vi "Toma_A.vi"() -> ()   [LabVIEW 2017]
uses:
  Maquina_de_Estados_Type_Def.ctl
  Cluster_de_Datos.ctl
  <vilib>/DAQmx/read.llb/DAQmx Read (Analog 1D DBL 1Chan NSamp).vi
  <vilib>/DAQmx/create/channels.llb/DAQmx Create Channel (AI-Voltage-Basic).vi
  <vilib>/DAQmx/configure/timing.llb/DAQmx Timing (Sample Clock).vi
  <vilib>/DAQmx/miscellaneous.llb/DAQmx Fill In Error Info.vi
  <vilib>/imath/engines/lvmath2/RunTimeEngine/BuiltInFunctions/length/NIMS_length(GV).vi
  <instcachedir>/0/NIMS_length(GV)_08A3D13377FD4E4B96F5795FBF3698FA.lvgen/NIMS_length(GV)_08A3D13377FD4E4B96F5795FBF3698FA_000.vi
  <vilib>/imath/engines/lvmath2/RunTimeEngine/IndexReplace/NIMS V(S)=S.vi
  <instcachedir>/0/NIMS V(S)=S_3F4D177D41884A9C969E5FA0B22E4B28.lvgen/NIMS V(S)=S_3F4D177D41884A9C969E5FA0B22E4B28_003.vi
  <vilib>/imathl/engines/lvmath/Functions/Error Handling/Create Error.vi
  <vilib>/imath/engines/lvmath2/RunTimeEngine/RangeToken/NIMS_Range_R2 - Integer.vi
  <instcachedir>/0/NIMS_Range_R2 - Integer_B2C3C6B11D0E4F789E1772ACB483EB02.lvgen/NIMS_Range_R2 - Integer_B2C3C6B11D0E4F789E1772ACB483EB02_000.vi
  <vilib>/imath/engines/lvmath2/RunTimeEngine/CommandStatement/MC_CommandStatement_break.vi
  <vilib>/imath/engines/lvmath2/RunTimeEngine/IndexRead/NIMS V(S).vi
  <instcachedir>/0/NIMS V(S)_0488751826AF41519A22953C041130DC.lvgen/NIMS V(S)_0488751826AF41519A22953C041130DC_000.vi
  <instcachedir>/0/NIMS V(S)=S_3F4D177D41884A9C969E5FA0B22E4B28.lvgen/NIMS V(S)=S_3F4D177D41884A9C969E5FA0B22E4B28_000.vi
  <vilib>/imath/engines/lvmath2/RunTimeEngine/ErrorHandling/NIMS_Create Error From Enums.vi
  <vilib>/imath/engines/lvmath2/RunTimeEngine/NodeEndStatement/NIMS_NodeEndStatement_Output.vi
  <instcachedir>/0/NIMS_NodeEndStatement_Output_53EC0D466D134D7ABD903AC30B43404B.lvgen/NIMS_NodeEndStatement_Output_53EC0D466D134D7ABD903AC30B43404B_005.vi
  <vilib>/imath/engines/lvmath2/RunTimeEngine/ErrorHandling/NIMS_Finalize Error.vi
  <vilib>/addons/_office/excel.llb/Excel Get Data (i32).vi
  <vilib>/addons/_office/excel.llb/Excel Easy Table (num).vi
  <vilib>/Utility/NIReport.llb/NI_report.lvclass
  <vilib>/Utility/NIReport.llb/Excel/NI_Excel.lvclass
  <vilib>/addons/_office/NI_ReportGenerationToolkit.lvlib
panel:
  in  "Ruta del Reporte":path
  in  "Ruta_Logo_IPN":path
  in  "Ruta_Logo_Upiita":path=path "C:/Users/LuisFernando/Documents/UPIITA/8vo semestre/Instrumentacion Virtual Aplicada/DAQ/Logo_Upiita.bmp"
  in  "Actualizar Rutas":bool
  in  "Calificacion":dbl
  in  "Grupo":string
  in  "Unidad de Aprendizaje":string
  in  "Leer Senal":bool
  in  "stop":bool
  in  "Comentarios":string
  out "Hora":string
  out "Fecha":string
  in  "Nombre (s):":string(combo)
  in  "Tab Control":enum32{"Función", "Derivada", "Integral"}(tab)
  out "Señal de Entrada M":dbl[](graph)
  out "Señal de Entrada":cluster{dbl[], "data":dbl[]}(graph)
  out "Derivada M":dbl[](graph)
  out "Derivada":cluster{"Tiempo":dbl[], "Diff":dbl[]}(graph)
  out "Integral M":dbl[](graph)
  out "Integral":cluster{"Tiempo":dbl[], "Integral":dbl[]}(graph)
  out "Escudo 2":picture
  out "Escudo_1":picture
  # "INSTITUTO POLITECNICO NACIONAL"
  # "Unidad Profesional Interdisciplinaria en\nIngenieria y Tecnologias Avanzadas"
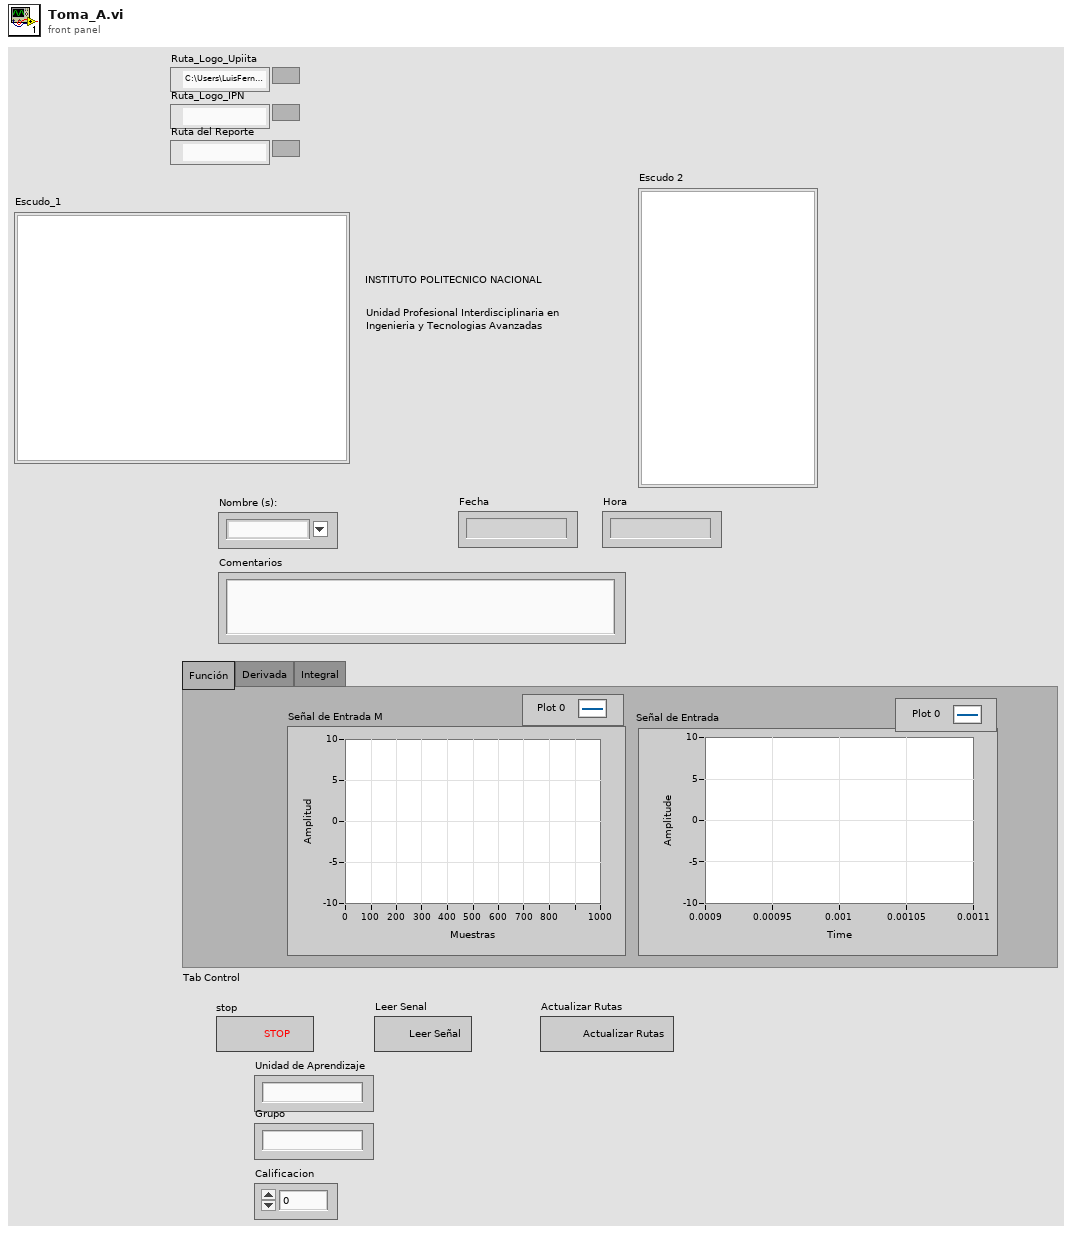
[diagram p1: front panel]
types:
  T1 = typedef "Cluster_de_Datos.ctl" = cluster{"Error":errorcluster, "Ruta_Logo_Upiita":path, "Ruta_Logo_IPN":path, "Señal de Entrada":dbl[], "Derivada":dbl[], "Integral":dbl[], "Muestras":i32, "Frecuencia de Muestreo":dbl, "Tiempo":dbl[], "dt":dbl, "Ruta del Reporte":path, "Numero de Hoja":u32}
  T2 = typedef "Maquina_de_Estados_Type_Def.ctl" = enum16{"Configuracion Inicial", "Espera", "Leer Senal", "Derivar", "Integrar", "Leer Datos de Usuario", "Salir"}
  T3 = enum16{"maximized", "minimized", "normal", "no change"}
  T4 = enum16{"Standard Report", "HTML", "Word", "Excel"}
  T5 = typedef "imagedata.ctl" = cluster{"image type":i32, "image depth":i32, "image":u8[], "mask":u8[], "colors":u32[], "Rectangle":cluster{"left":i16, "top":i16, "right":i16, "bottom":i16}}
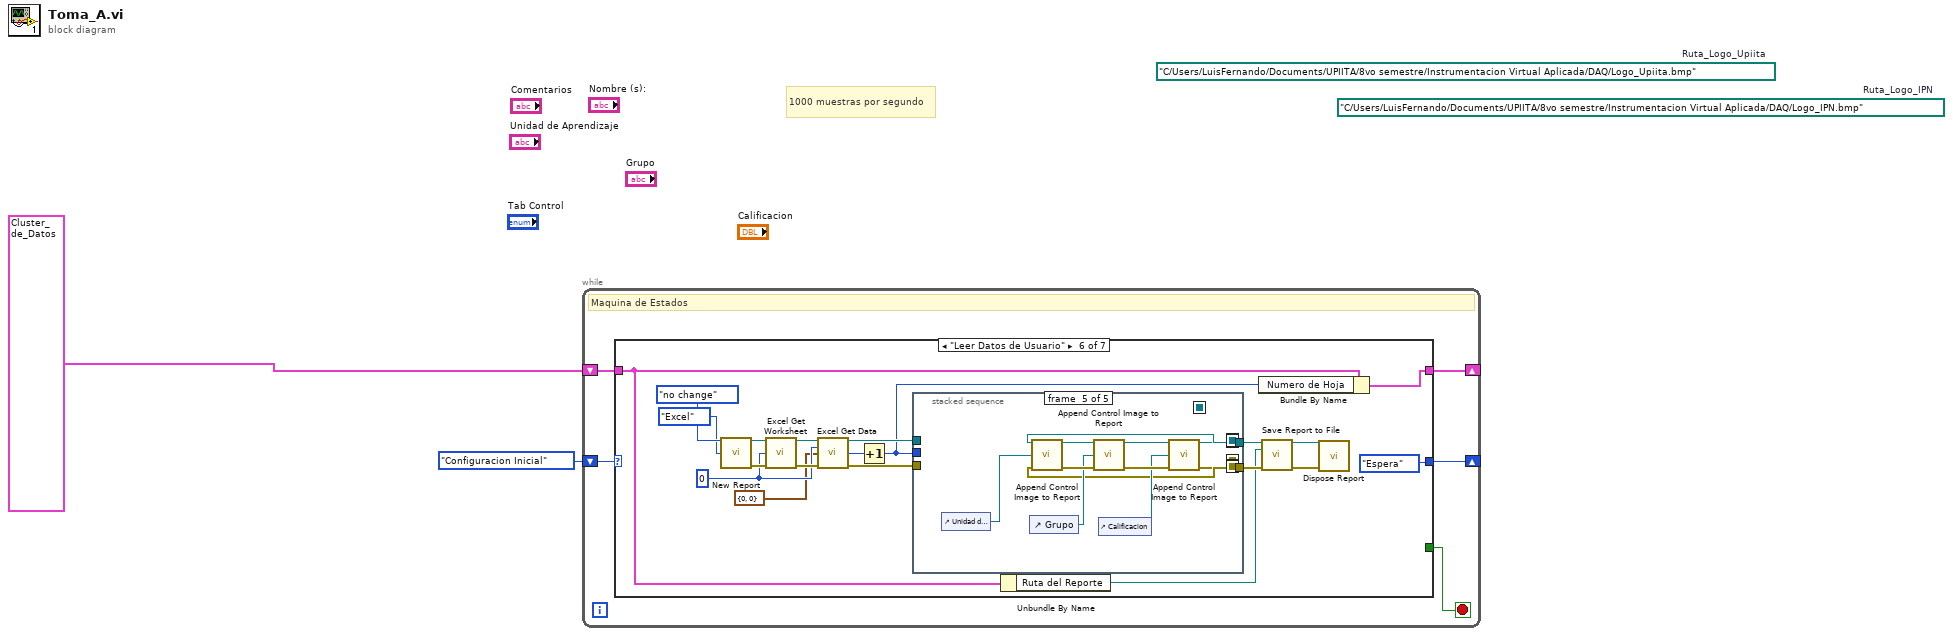
[diagram p0: block diagram]
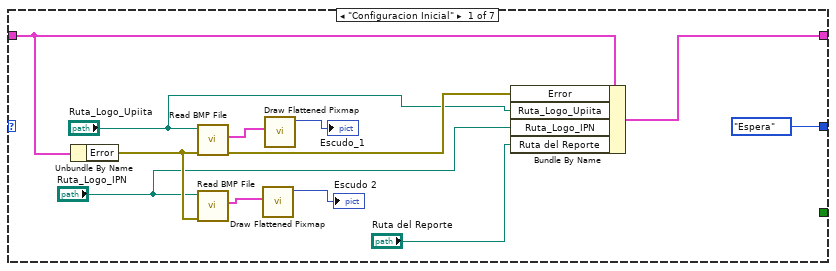
[diagram p2: hidden frame]
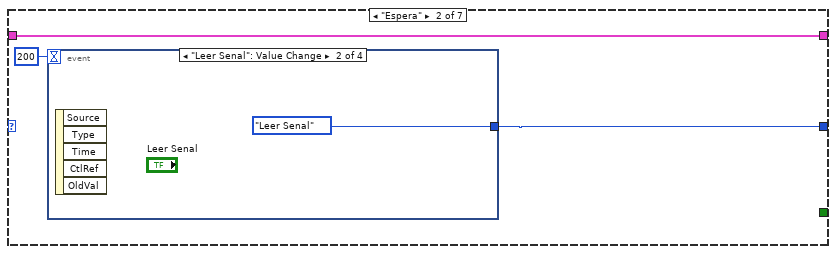
[diagram p3: hidden frame]
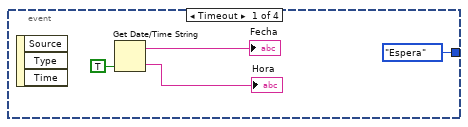
[diagram p4: hidden frame]
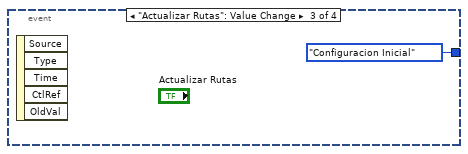
[diagram p5: hidden frame]
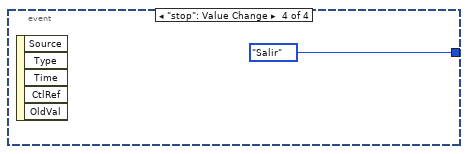
[diagram p6: hidden frame]
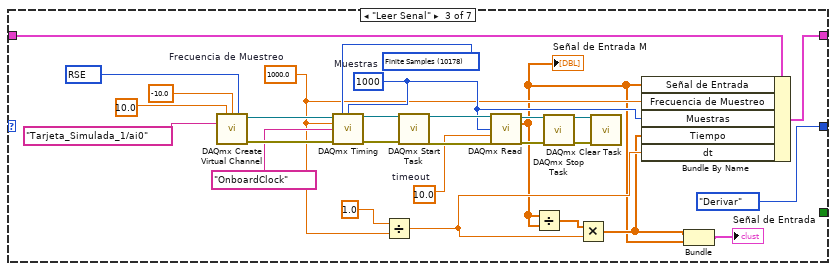
[diagram p7: hidden frame]
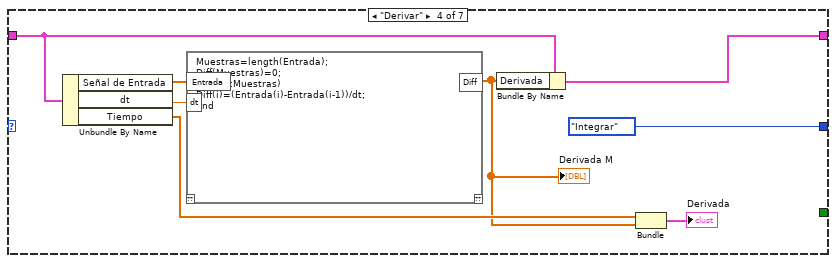
[diagram p8: hidden frame]
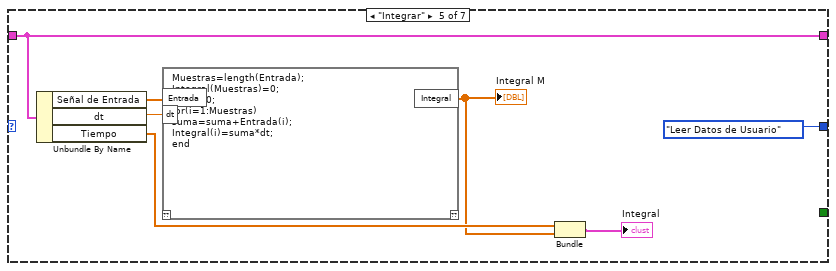
[diagram p9: hidden frame]
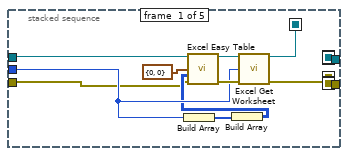
[diagram p10: hidden frame]
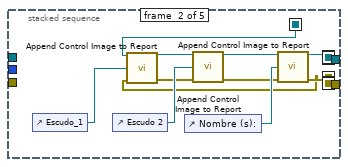
[diagram p11: hidden frame]
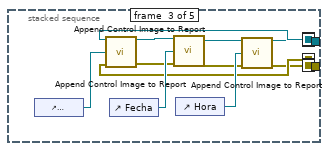
[diagram p12: hidden frame]
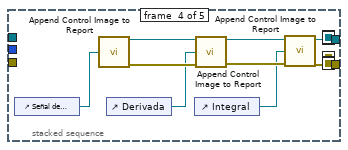
[diagram p13: hidden frame]
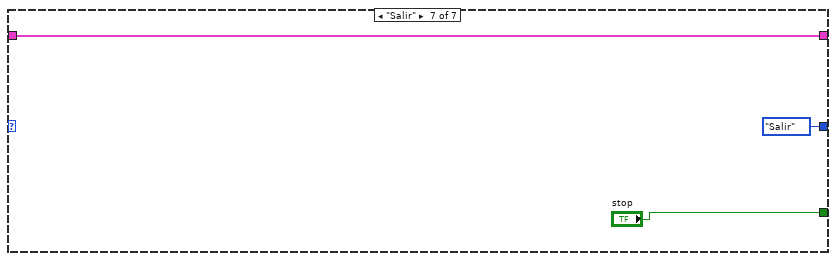
[diagram p14: hidden frame]
diagram:
  (unwired) path "C:/Users/LuisFernando/Documents/UPIITA/8vo semestre/Instrumentacion Virtual Aplicada/DAQ/Logo_IPN.bmp"  # Ruta_Logo_IPN
  (unwired) path "C:/Users/LuisFernando/Documents/UPIITA/8vo semestre/Instrumentacion Virtual Aplicada/DAQ/Logo_Upiita.bmp"  # Ruta_Logo_Upiita
  # "1000 muestras por segundo"
  n1 = while {
    shift-right: [w6] -> _
    shift-left: Maquina_de_Estados_Type_Def."Configuracion Inicial" -> [w7]
    shift-right: [w4] -> _
    shift-left: T1 {"Error"={"status"=FALSE, "code"=0, "source"=""}, "Ruta_Logo_Upiita"=path "C:/Users/LuisFernando/Documents/UPIITA/8vo semestre/Instrumentacion Virtual Aplicada/DAQ/Logo_Upiita.bmp", "Ruta_Logo_IPN"=path "C:/Users/LuisFernando/Documents/UPIITA/8vo semestre/Instrumentacion Virtual Aplicada/DAQ/Logo_IPN.bmp", "Señal de Entrada"=[], "Derivada"=[], "Integral"=[], "Muestras"=1000, "Frecuencia de Muestreo"=10.0, "Tiempo"=[], "dt"=1000.0, "Ruta del Reporte"=path "C:/Users/LuisFernando/Documents/UPIITA/8vo semestre/Instrumentacion Virtual Aplicada/DAQ/Logo_IPN.bmp", "Numero de Hoja"=0} -> [w5]
    stop <- w3 stop-if-true
    # "Maquina de Estados"
    n2 = case shown="\"Leer Datos de Usuario\"" w7 {
      tunnel: [Maquina_de_Estados_Type_Def."Espera" w21 Maquina_de_Estados_Type_Def."Derivar" Maquina_de_Estados_Type_Def."Integrar" Maquina_de_Estados_Type_Def."Leer Datos de Usuario" Maquina_de_Estados_Type_Def."Espera" Maquina_de_Estados_Type_Def."Salir"] -> w6
      tunnel: w5 -> [w15 w22 w39 w63 w182 w318 w393]
      tunnel: [w17 w22 w38 w62 w182 w335 w393] -> w4
      tunnel: [_ _ _ _ _ _ "stop"] -> w3
      frame "Configuracion Inicial" {
        n3 = Unbundle By Name(w15) -> ("Error"=w13:errorcluster)
        n4 = call <vilib>:"Read BMP File.vi"("error in (no error)"=w13, "path to BMP file"="Ruta_Logo_Upiita") -> ("error out"=w16:errorcluster, "image data"=w18:T5)  [unwired: 7 in, 1 out]
        n5 = call <vilib>:"Read BMP File.vi"("error in (no error)"=w13, "path to BMP file"="Ruta_Logo_IPN") -> ("image data"=w14:T5)  [unwired: 7 in, 2 out]
        n6 = call <vilib>:"Draw Flattened Pixmap.vi"("image data"=w14) -> ("new picture"=→"Escudo 2":picture)  [unwired: 8 in]
        n7 = call <vilib>:"Draw Flattened Pixmap.vi"("image data"=w18) -> ("new picture"=→"Escudo_1":picture)  [unwired: 8 in]
        n8 = Bundle By Name(cluster=w15, "Error"=w16, "Ruta_Logo_Upiita"="Ruta_Logo_Upiita", "Ruta_Logo_IPN"="Ruta_Logo_IPN", "Ruta del Reporte"="Ruta del Reporte") -> (w17:T1)
      }
      frame "Espera" {
        n9 = event shown="[1] \"Leer Senal\": Value Change" {
          selector: _ -> [_ _ _ _]
          dyn-events: _ -> [_ _ _ _]
          timeout: 200 -> [_ _ _ _]
          tunnel: [Maquina_de_Estados_Type_Def."Espera" Maquina_de_Estados_Type_Def."Leer Senal" Maquina_de_Estados_Type_Def."Configuracion Inicial" Maquina_de_Estados_Type_Def."Salir"] -> w21
          event Timeout {
            n10 = event-data() -> ()  [unwired: 1 in, 3 out]
            n11 = Get Date/Time String(want seconds? (F)=TRUE) -> (date string=→"Fecha":string, time string=→"Hora":string)  [unwired: 2 in]
          }
          event "Leer Senal": Value Change {
            n12 = event-data() -> ()  [unwired: 1 in, 5 out]
          }
          event "Actualizar Rutas": Value Change {
            n13 = event-data() -> ()  [unwired: 1 in, 5 out]
          }
          event "stop": Value Change {
            n14 = event-data() -> ()  [unwired: 1 in, 5 out]
          }
        }
      }
      frame "Leer Senal" {
        w46 = 10.0  # timeout
        w41 = 10083 items=["Default"=-1, "RSE"=10083, "NRSE"=10078, "Differential"=10106, "Pseudodifferential"=12529] ("input terminal configuration")
        w35 = 1000.0  # Frecuencia de Muestreo
        w37 = 1000  # Muestras
        w45 = 10178 items=["Finite Samples"=10178, "Continuous Samples"=10123, "Hardware Timed Single Point"=12522] ("sample mode")
        n15 = call-poly <vilib>:"DAQmx Create Virtual Channel.vi"("maximum value"=10.0, "minimum value"=-10.0, "input terminal configuration"=w41, "physical channels"=tag "Tarjeta_Simulada_1/ai0") -> ("task out"=w48:refnum<k21>, "error out"=w47:errorcluster)  [unwired: 10 in]
        n16 = call-poly <vilib>:"DAQmx Timing.vi"("task/channels in"=w48, "sample mode"=w45, "samples per channel"=w37, "rate"=w35, "source"=tag "OnboardClock", "error in"=w47) -> ("task out"=w49:refnum<k21>, "error out"=w50:errorcluster)  [unwired: 8 in]
        n17 = Divide(x=1.0, y=w35) -> (x/y=w33:dbl)
        n18 = call <vilib>:"DAQmx Start Task.vi"("task/channels in"=w49, "error in"=w50) -> ("task out"=w51:refnum<k21>, "error out"=w52:errorcluster)  [unwired: 12 in]
        n19 = call-poly <vilib>:"DAQmx Read.vi"("task/channels in"=w51, "number of samples per channel"=w37, "timeout"=w46, "error in"=w52) -> ("task out"=w53:refnum<k21>, "data"=w31:dbl[], "error out"=w54:errorcluster)  [unwired: 9 in]
        "Señal de Entrada M" <- w31
        n20 = Divide(x=w31, y=w31) -> (x/y=w34:dbl[])
        n21 = call <vilib>:"DAQmx Stop Task.vi"("task/channels in"=w53, "error in"=w54) -> ("task out"=w55:refnum<k21>, "error out"=w56:errorcluster)  [unwired: 12 in]
        n22 = Multiply(x=w34, y=w33) -> (x*y=w32:dbl[])
        n23 = call <vilib>:"DAQmx Clear Task.vi"("task in"=w55, "error in"=w56) -> ()  [unwired: 13 in, 1 out]
        n24 = Bundle By Name(cluster=w39, "Señal de Entrada"=w31, "Frecuencia de Muestreo"=w35, "Muestras"=w37, "Tiempo"=w32, "dt"=w33) -> (w38:T1)
        n25 = Bundle(w32, "data"=w31) -> (→"Señal de Entrada":cluster{dbl[], "data":dbl[]})  [unwired: 1 in]
      }
      frame "Derivar" {
        n26 = Unbundle By Name(w63) -> ("Señal de Entrada"=w64:dbl[], "dt"=w61:dbl, "Tiempo"=w59:dbl[])
        n27 = mathscript code="Muestras=length(Entrada);\nDiff(Muestras)=0;\nfor(i=2:Muestras)\nDiff(i)=(Entrada(i)-Entrada(i-1))/dt;\nend"("Entrada"=w64, "dt"=w61) -> ("Diff"=w58:dbl[])  [unwired: 1 in, 1 out]
        "Derivada M" <- w58
        n28 = Bundle By Name(cluster=w63, "Derivada"=w58) -> (w62:T1)
        n29 = Bundle("Tiempo"=w59, "Diff"=w58) -> (→"Derivada":cluster{"Tiempo":dbl[], "Diff":dbl[]})  [unwired: 1 in]
      }
      frame "Integrar" {
        n30 = Unbundle By Name(w182) -> ("Señal de Entrada"=w181:dbl[], "dt"=w180:dbl, "Tiempo"=w179:dbl[])
        n31 = mathscript code="Muestras=length(Entrada);\nIntegral(Muestras)=0;\nsuma=0;\nfor(i=1:Muestras)\nsuma=suma+Entrada(i);\nIntegral(i)=suma*dt;\nend"("Entrada"=w181, "dt"=w180) -> ("Integral"=w177:dbl[])  [unwired: 1 in, 1 out]
        "Integral M" <- w177
        n32 = Bundle("Tiempo"=w179, "Integral"=w177) -> (→"Integral":cluster{"Tiempo":dbl[], "Integral":dbl[]})  [unwired: 1 in]
      }
      frame "Leer Datos de Usuario" {
        w323 = 0 ("worksheet index (0)")
        n33 = call <vilib>:"New Report.vi"("window state (normal)"=T3."no change", "report type"=T4."Excel") -> ("report out"=w332:refnum<class "NI_report.lvclass">, "error out"=w331:errorcluster)  [unwired: 12 in]
        n34 = call <vilib>:"Excel Get Worksheet.vi"("report in"=w332, "worksheet index (0)"=w323, "error in (no error)"=w331) -> ("report out"=w330:refnum<class "NI_report.lvclass">, "error out"=w329:errorcluster)  [unwired: 11 in]
        n35 = call-poly <vilib>:"Excel Get Data.vi"("report in"=w330, "data type"=w323, "start (0, 0)"=cluster{"start row":i32, "start column":i32} {"start row"=0, "start column"=0}, "error in (no error)"=w329) -> ("report out"=w333:refnum<class "NI_report.lvclass">, "data"=w328:i32, "error out"=w334:errorcluster)  [unwired: 9 in]
        n36 = Increment(x=w328) -> (x+1=w319:i32)
        n37 = stacked-sequence {
          seq-local: [w344 _ _ _ _] -> [_ w348 _ _ _]
          seq-local: [w343 _ _ _ _] -> [_ w347 _ _ _]
          seq-local: [_ w350 _ _ _] -> [_ _ w361 _ _]
          seq-local: [_ w349 _ _ _] -> [_ _ w360 _ _]
          seq-local: [_ _ w359 _ _] -> [_ _ _ w372 _]
          seq-local: [_ _ w358 _ _] -> [_ _ _ w371 _]
          seq-local: [_ _ _ w370 _] -> [_ _ _ _ w383]
          seq-local: [_ _ _ w369 _] -> [_ _ _ _ w382]
          tunnel: w319 -> [w342 _ _ _ _]
          tunnel: w333 -> [w338 _ _ _ _]
          tunnel: w334 -> [w337 _ _ _ _]
          tunnel: [_ _ _ _ w381] -> w327
          tunnel: [_ _ _ _ w380] -> w326
          frame #0 {
            n38 = Build Array(w342) -> (w340:i32[])
            n39 = Build Array(w340) -> (w339:i32[][])
            n40 = call-poly <vilib>:"Excel Easy Table.vi"("report in"=w338, "start (0, 0)"=cluster{"start row":i32, "start column":i32} {"start row"=0, "start column"=0}, "text data"=w339, "error in (no error)"=w337) -> ("report out"=w345:refnum<class "NI_report.lvclass">, "error out"=w346:errorcluster)  [unwired: 7 in, 3 out]
            n41 = call <vilib>:"Excel Get Worksheet.vi"("report in"=w345, "worksheet index (0)"=w342, "error in (no error)"=w346) -> ("report out"=w344:refnum<class "NI_report.lvclass">, "error out"=w343:errorcluster)  [unwired: 11 in]
          }
          frame #1 {
            n42 = control-ref of="Escudo_1"() -> (w351:refnum<vi>)
            n43 = control-ref of="Escudo 2"() -> (w354:refnum<vi>)
            n44 = call-dynamic "Append Control Image to Report.vi"("report in"=w348, "ctrl reference"=w351, "error in (no error)"=w347) -> ("report out"=w352:refnum<class "NI_report.lvclass">, "error out"=w353:errorcluster)  [unwired: 9 in, 2 out]
            n45 = control-ref of="Nombre (s):"() -> (w357:refnum<vi>)
            n46 = call-dynamic "Append Control Image to Report.vi"("report in"=w352, "ctrl reference"=w354, "error in (no error)"=w353) -> ("report out"=w355:refnum<class "NI_report.lvclass">, "error out"=w356:errorcluster)  [unwired: 9 in, 2 out]
            n47 = call-dynamic "Append Control Image to Report.vi"("report in"=w355, "ctrl reference"=w357, "error in (no error)"=w356) -> ("report out"=w349:refnum<class "NI_report.lvclass">, "error out"=w350:errorcluster)  [unwired: 9 in, 2 out]
          }
          frame #2 {
            n48 = control-ref of="Comentarios"() -> (w362:refnum<vi>)
            n49 = call-dynamic "Append Control Image to Report.vi"("report in"=w360, "ctrl reference"=w362, "error in (no error)"=w361) -> ("report out"=w364:refnum<class "NI_report.lvclass">, "error out"=w363:errorcluster)  [unwired: 9 in, 2 out]
            n50 = control-ref of="Fecha"() -> (w365:refnum<vi>)
            n51 = call-dynamic "Append Control Image to Report.vi"("report in"=w364, "ctrl reference"=w365, "error in (no error)"=w363) -> ("report out"=w367:refnum<class "NI_report.lvclass">, "error out"=w366:errorcluster)  [unwired: 9 in, 2 out]
            n52 = control-ref of="Hora"() -> (w368:refnum<vi>)
            n53 = call-dynamic "Append Control Image to Report.vi"("report in"=w367, "ctrl reference"=w368, "error in (no error)"=w366) -> ("report out"=w359:refnum<class "NI_report.lvclass">, "error out"=w358:errorcluster)  [unwired: 9 in, 2 out]
          }
          frame #3 {
            n54 = control-ref of="Señal de Entrada"() -> (w373:refnum<vi>)
            n55 = call-dynamic "Append Control Image to Report.vi"("report in"=w372, "ctrl reference"=w373, "error in (no error)"=w371) -> ("report out"=w379:refnum<class "NI_report.lvclass">, "error out"=w377:errorcluster)  [unwired: 9 in, 2 out]
            n56 = control-ref of="Derivada"() -> (w374:refnum<vi>)
            n57 = control-ref of="Integral"() -> (w375:refnum<vi>)
            n58 = call-dynamic "Append Control Image to Report.vi"("report in"=w379, "ctrl reference"=w374, "error in (no error)"=w377) -> ("report out"=w378:refnum<class "NI_report.lvclass">, "error out"=w376:errorcluster)  [unwired: 9 in, 2 out]
            n59 = call-dynamic "Append Control Image to Report.vi"("report in"=w378, "ctrl reference"=w375, "error in (no error)"=w376) -> ("report out"=w369:refnum<class "NI_report.lvclass">, "error out"=w370:errorcluster)  [unwired: 9 in, 2 out]
          }
          frame #4 {
            n60 = control-ref of="Unidad de Aprendizaje"() -> (w384:refnum<vi>)
            n61 = control-ref of="Grupo"() -> (w385:refnum<vi>)
            n62 = call-dynamic "Append Control Image to Report.vi"("report in"=w382, "ctrl reference"=w384, "error in (no error)"=w383) -> ("report out"=w387:refnum<class "NI_report.lvclass">, "error out"=w388:errorcluster)  [unwired: 9 in, 2 out]
            n63 = call-dynamic "Append Control Image to Report.vi"("report in"=w387, "ctrl reference"=w385, "error in (no error)"=w388) -> ("report out"=w389:refnum<class "NI_report.lvclass">, "error out"=w390:errorcluster)  [unwired: 9 in, 2 out]
            n64 = control-ref of="Calificacion"() -> (w386:refnum<vi>)
            n65 = call-dynamic "Append Control Image to Report.vi"("report in"=w389, "ctrl reference"=w386, "error in (no error)"=w390) -> ("report out"=w381:refnum<class "NI_report.lvclass">, "error out"=w380:errorcluster)  [unwired: 9 in, 2 out]
          }
        }
        n66 = Unbundle By Name(w318) -> ("Ruta del Reporte"=w317:path)
        n67 = Bundle By Name(cluster=w318, "Numero de Hoja"=w319) -> (w335:T1)
        n68 = call-dynamic "Save Report to File.vi"("report in"=w327, "report file path"=w317, "error in (no error)"=w326) -> ("report out"=w325:refnum<class "NI_report.lvclass">, "error out"=w324:errorcluster)  [unwired: 11 in]
        n69 = call-dynamic "Dispose Report.vi"("report in"=w325, "error in (no error)"=w324) -> ()  [unwired: 13 in, 1 out]
      }
      frame "Salir" {
      }
    }
  }
